vi "DDS - Pulse.vi"(7 "Reset Accumulator":bool, 9 "Pulse Number":enum16{"Single Pulse", "Two Pulse"}(ring), 10 "Accumulator Increment":fxp<+,32,32>) -> (1 "Accumulator Value":fxp<+,32,32>, 2 "data out":i16 caption="Data Out")   [LabVIEW 2015]
uses:
  <vilib>/rvi/FXPMathLib/FxpAdd/XNode/nifxpmath_Add.xnode
  <vilib>/rvi/FXPMathLib/sim/FxpSim.dll
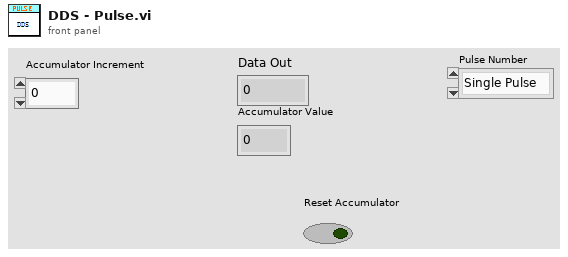
[diagram p1: front panel]
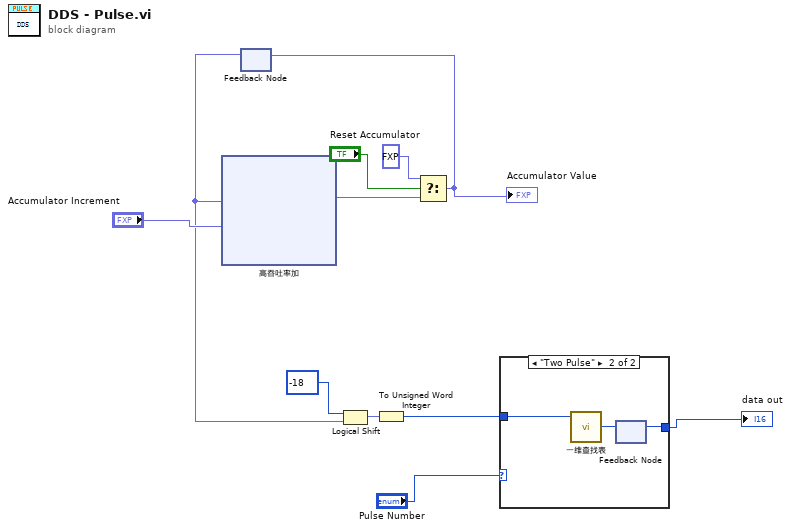
[diagram p0: block diagram]
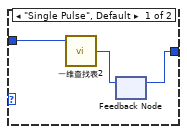
[diagram p2: hidden frame]
diagram:
  n1 = feedback #1() -> (w3:fxp<+,32,32>)  [unwired: 1 in]
  n2 = xnode ("高吞吐率加")("x"=w3, "y"="Accumulator Increment") -> ("x+y"=w9:fxp<+,32,32>)
  n3 = Logical Shift(y=i16 -18, x=w3) -> (x << y=w5:fxp<+,32,32>)
  n4 = To Unsigned Word Integer(number=w5) -> (unsigned 16bit integer=w4:u16)
  n5 = Select(t=fxp<+,32,32> 0.0, s="Reset Accumulator", f=w9) -> (s? t:f=w10:fxp<+,32,32>)
  "Accumulator Value" <- w10
  n6 = feedback-in #1(w10) -> ()
  n7 = case shown="\"Two Pulse\"" "Pulse Number" {
    tunnel: [w12 w16] -> w1
    tunnel: w4 -> [w14 w17]
    frame "Single Pulse", Default {
      n8 = call "一维查找表2"("address"=w14) -> ("data out"=w13:i16)  [unwired: 8 in]
      n9 = feedback #2 ("反馈节点")() -> (w12:i16)  [unwired: 1 in]
      n10 = feedback-in #2(w13) -> ()
    }
    frame "Two Pulse" {
      n11 = call "一维查找表"("address"=w17) -> ("data out"=w15:i16)  [unwired: 8 in]
      n12 = feedback #3 ("反馈节点")() -> (w16:i16)  [unwired: 1 in]
      n13 = feedback-in #3(w15) -> ()
    }
  }
  "data out" <- w1
